vi "Network Shared Variable Check.vi"() -> ()   [LabVIEW 2013]
panel:
  in  "stop":bool
  out "PS2Voltage":dbl
  in  "PS1Voltage":dbl
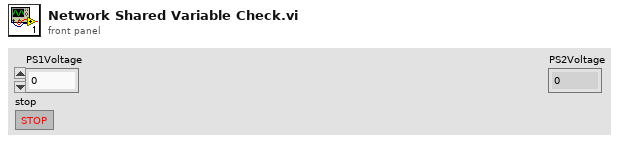
[diagram p1: front panel]
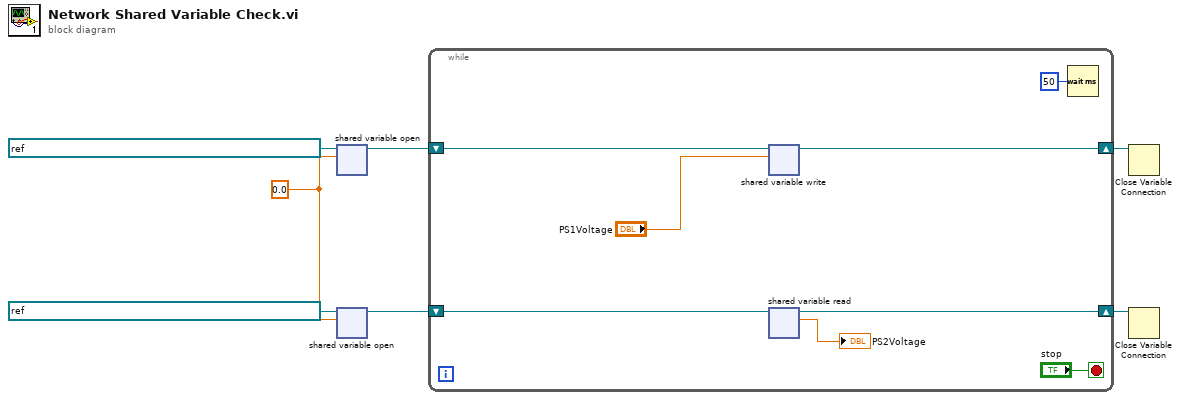
[diagram p0: block diagram]
diagram:
  w1 = 0.0
  n1 = shared-variable-open(refnum<k21> "ni.var.psp://rt single-board rio/PS Control/PS1Voltage" ("shared variable refnum in"), w1) -> (w5:refnum<k21>)  [unwired: 2 in, 1 out]
  n2 = shared-variable-open(refnum<k21> "ni.var.psp://rt single-board rio/PS Control/PS2Voltage" ("shared variable refnum in"), w1) -> (w4:refnum<k21>)  [unwired: 2 in, 1 out]
  n3 = while {
    shift-right: [w10] -> w3
    shift-left: w4 -> [w11]
    shift-right: [w12] -> w2
    shift-left: w5 -> [w13]
    stop <- "stop" stop-if-true
    n4 = shared-variable-write(w13, "PS1Voltage") -> (w12:refnum<k21>)  [unwired: 1 in, 1 out]
    n5 = shared-variable-read(w11) -> (w10:refnum<k21>, →"PS2Voltage":dbl)  [unwired: 1 in, 2 out]
    n6 = Wait (ms)(milliseconds to wait=u32 50) -> ()  [unwired: 1 out]
  }
  n7 = Close Variable Connection(11:w2) -> ()  [unwired: 1 in, 1 out]
  n8 = Close Variable Connection(11:w3) -> ()  [unwired: 1 in, 1 out]
